vi "add1.vi"() -> ()   [LabVIEW 2020]
panel:
  out "a+b":dbl
  in  "b":dbl
  in  "a":dbl
  out "cm":string
  in  "路径":path
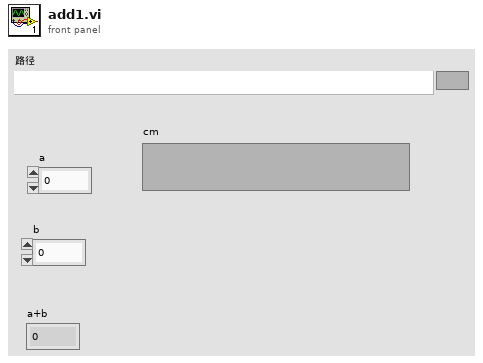
[diagram p1: front panel]
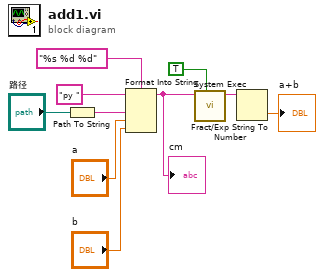
[diagram p0: block diagram]
diagram:
  n1 = Path To String(path="路径") -> (string=w9:string)
  n2 = Format Into String(format string="%s %d %d" ("格式字符串"), initial string="py ", w9, "a", "b") -> (resulting string=w2:string)  [unwired: 1 in, 1 out]
  "cm" <- w2
  n3 = call <vilib>:"System Exec.vi"("wait until completion? (T)"=TRUE, "command line"=w2) -> ("standard output"=w5:string)  [unwired: 6 in, 3 out]
  n4 = Fract/Exp String To Number(string=w5) -> (number=→"a+b":dbl)  [unwired: 3 in, 1 out]
